vi "Load_from_Project.vi"(6 "commonPath":path, 8 "error in (no error)":errorcluster, 9 "index":i32, 10 "buildObject":T1, 11 "AB_Destination in":refnum<class "AB_Destination.lvclass">) -> (0 "error out":errorcluster, 3 "AB_Destination out":refnum<class "AB_Destination.lvclass">)   [LabVIEW 2020, in "AB_Destination.lvclass"]
uses:
  <vilib>/AppBuilder/AB_Classes/Destination/AB_Destination.lvclass
  <resource>/Framework/Providers/API/ItemRef.ctl
  <vilib>/AppBuilder/RW_Project/AB_RW_Project_PropBag_Action.ctl
  <vilib>/AppBuilder/AB_Classes/Destination/AB_Destination.lvclass/AB_Destination.ctl
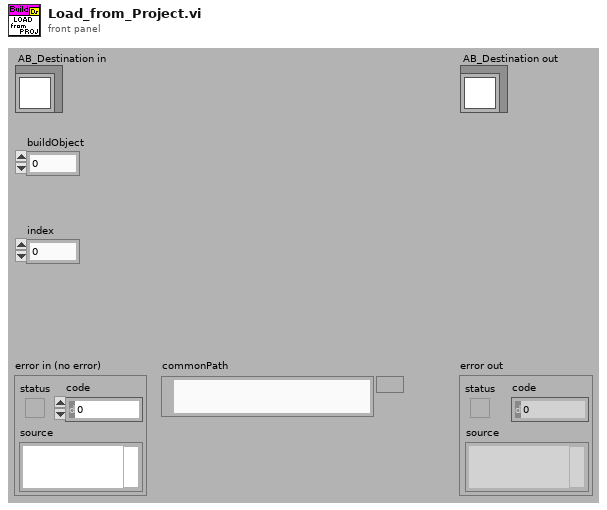
[diagram p1: front panel]
types:
  T1 = typedef "ItemRef.ctl" = u64
  T2 = typedef "AB_RW_Project_PropBag_Action.ctl" = enum16{"read", "write", "clear", "readPrevious", "writePrevious", "clearPrevious"}
  T3 = typedef "AB_RW_Project_Destination_Data.ctl" = cluster{"destName":string, "path":path, "preserveHierarchy":bool, "libraryName":string}
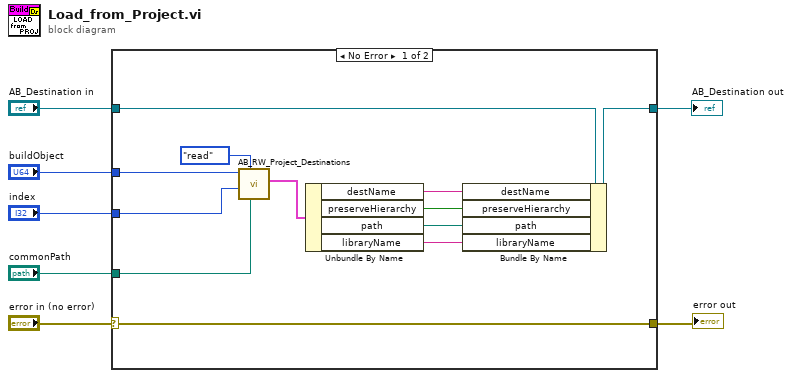
[diagram p0: block diagram]
diagram:
  n1 = case shown="No Error" "error in (no error)" {
    selector: "error in (no error)" -> [w19 w21]
    tunnel: [w19 w21] -> w6
    tunnel: [w17 w20] -> w4
    tunnel: "AB_Destination in" -> [w18 w20]
    tunnel: "buildObject" -> [w16 _]
    tunnel: "index" -> [w14 _]
    tunnel: "commonPath" -> [w9 _]
    frame No Error {
      n2 = call <vilib>:"AB_RW_Project_Destinations.vi"("ProjectPath"=w9, "action"=AB_RW_Project_PropBag_Action."read", "index"=w14, "buildObject"=w16) -> ("data out"=w13:T3)  [unwired: 2 in, 5 out]
      n3 = Unbundle By Name(w13) -> ("destName"=w12:string, "preserveHierarchy"=w11:bool, "path"=w10:path, "libraryName"=w8:string)
      n4 = Bundle By Name(cluster=w18, "destName"=w12, "preserveHierarchy"=w11, "path"=w10, "libraryName"=w8) -> (w17:refnum<class "AB_Destination.lvclass">)
    }
    frame Error {
    }
  }
  "error out" <- w6
  "AB_Destination out" <- w4
